vi "Configure Modulation (FSK).vi"(0 "VISA resource name":refnum<visa-resource-name>, 1 "Enable FSK Modulation (T:Enable)":bool=TRUE, 5 "FSK Source (0: Internal)":u16(ring) items=["Internal", "External"], 7 "Channel (1:Channel 1)":i32(ring)=1 items=["Channel 1"=1, "Channel 2"=2], 9 "Hop Frequency (100.000 Hz)":dbl=100.0 format="%.3f", 11 "error in (no error)":errorcluster, 12 "Key Frequency (100.000 Hz)":dbl=100.0 format="%.3f") -> (4 "VISA resource name out":refnum<visa-resource-name>, 15 "error out":errorcluster)   [LabVIEW 2023, in "Siglent SDG X Series.lvlib"]
doc: "Configures and enables FSK modulation.\n\n<B>Note:</B> The carrier waveform shape and parameters are set by the Configure Standard Waveform VI."
uses:
  Siglent SDG X Series.lvlib
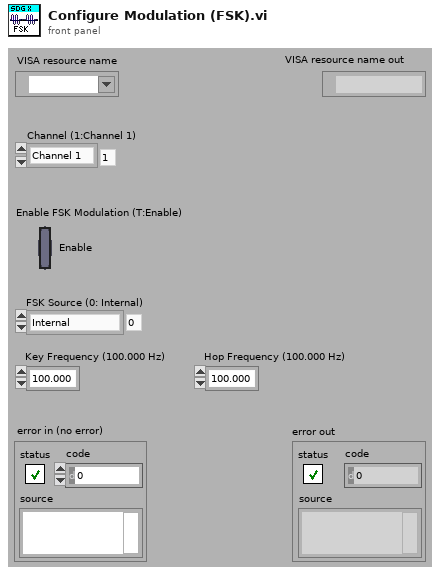
[diagram p1: front panel]
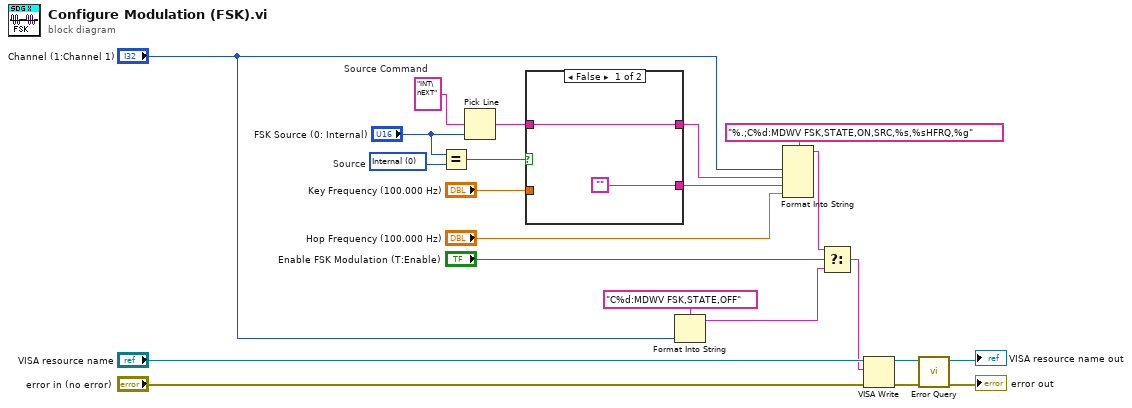
[diagram p0: block diagram]
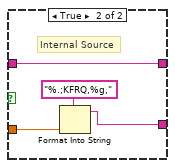
[diagram p2: hidden frame]
diagram:
  w15 = "INT\nEXT"  # Source Command
  w11 = u16 0 items=["Internal", "External"]  # Source
  n1 = Equal?(x="FSK Source (0: Internal)", y=w11) -> (x = y?=w14:bool)
  n2 = Pick Line(multi-line string=w15, line index="FSK Source (0: Internal)") -> (output string=w13:string)  [unwired: 1 in]
  n3 = case shown="False" w14 {
    tunnel: w13 -> [w24 w28]
    tunnel: [w24 w28] -> w9
    tunnel: ["" w25] -> w7
    tunnel: "Key Frequency (100.000 Hz)" -> [_ w26]
    frame False {
    }
    frame True {
      # "Internal Source"
      n4 = Format Into String(format string="%.;KFRQ,%g,", w26) -> (resulting string=w25:string)  [unwired: 2 in, 1 out]
    }
  }
  n5 = Format Into String(format string="C%d:MDWV FSK,STATE,OFF", "Channel (1:Channel 1)") -> (resulting string=w4:string)  [unwired: 2 in, 1 out]
  n6 = Format Into String(format string="%.;C%d:MDWV FSK,STATE,ON,SRC,%s,%sHFRQ,%g", "Channel (1:Channel 1)", w9, w7, "Hop Frequency (100.000 Hz)") -> (resulting string=w3:string)  [unwired: 2 in, 1 out]
  n7 = Select(t=w3, s="Enable FSK Modulation (T:Enable)", f=w4) -> (s? t:f=w2:string)
  n8 = VISA Write(VISA resource name="VISA resource name", write buffer=w2, error in (no error)="error in (no error)") -> (VISA resource name out=w20:refnum<visa-resource-name>, error out=w19:errorcluster)  [unwired: 1 out]
  n9 = call "Error Query.vi"("error in (no error)"=w19, "VISA resource name"=w20) -> ("error out"=→"error out":errorcluster, "VISA resource name out"=→"VISA resource name out":refnum<visa-resource-name>)  [unwired: 6 in, 2 out]
